vi "generate default line.vi"(8 "error in":errorcluster, 10 "last line":T1, 11 "operations table":T2) -> (0 "error out":errorcluster, 2 "line":T1)   [LabVIEW 2013, in "Modbus Slave editor node.lvclass"]
doc: "Platypus Framework 1.0.1.65\nNI Systems Engineering - National Instruments"
uses:
  Modbus Slave editor node.lvclass
  table line.ctl
  <vilib>/NI/Tag Bus/tag/tag descriptor.lvclass
  module/module channel/Modbus Module Channel.lvclass
  <vilib>/NI/Tag Bus/tag/Data Type.ctl
  module/module channel/data bank type.ctl
  table reference.ctl
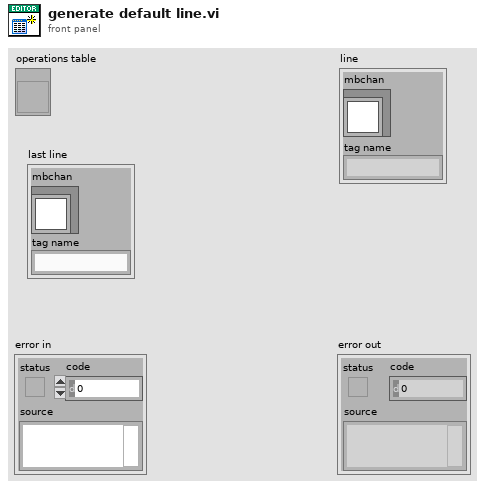
[diagram p1: front panel]
types:
  T1 = typedef "Modbus Slave editor node.lvclass/table line.ctl" = cluster{"mbchan":refnum<class "Modbus Module Channel.lvclass">, "tag name":string}
  T2 = typedef "Modbus Slave editor node.lvclass/table reference.ctl" = refnum<vi>
  T3 = typedef "tag bus.lvlib/tag descriptor.lvclass/Data Type.ctl" = enum16{"Double", "Single", "I64", "I32", "I16", "I8", "U64", "U32", "U16", "U8", "Boolean", "String", "Array of Double", "Array of Single", "Array of I64", "Array of I32", "Array of I16", "Array of I8", "Array of U64", "Array of U32", "Array of U16", "Array of U8", "Array of Boolean", "Array of String"}
  T4 = typedef "Modbus Module Channel.lvclass/data bank type.ctl" = enum16{"coils", "discrete inputs", "input registers", "holding registers"}
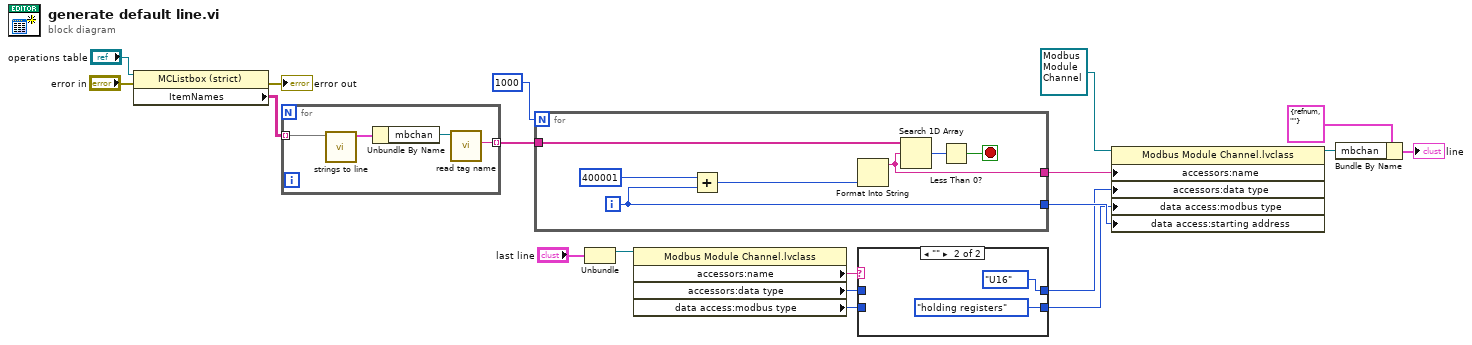
[diagram p0: block diagram]
diagram:
  n1 = property class="MCListbox (strict)"(reference="operations table", error in="error in") -> (error out=→"error out":errorcluster, "ItemNames"=w16:string[][])  [unwired: 1 out]
  n2 = for {
    tunnel: w16 -> [w23] mode=indexing
    tunnel: [w20] -> w14 mode=indexing
    n3 = call "strings to line.vi"("strings"=w23) -> ("line"=w22:T1)  [unwired: 10 in]
    n4 = Unbundle By Name(w22) -> ("mbchan"=w21:refnum<class "Modbus Module Channel.lvclass">)
    n5 = call <vilib>:"read tag name.vi"("system tag in"=w21) -> ("name"=w20:string)  [unwired: 8 in, 2 out]
  }
  n6 = for {
    N: 1000 -> [_]
    tunnel: w14 -> [w30]
    tunnel: [w27] -> w9
    tunnel: [w24] -> w8
    i -> [w24]
    stop <- w28 stop-if-true
    n7 = Add(x=400001, y=w24) -> (x+y=w26:i32)
    n8 = Format Into String(w26) -> (resulting string=w27:string)  [unwired: 3 in, 1 out]
    n9 = Search 1D Array(1D array=w30, element=w27) -> (index of element=w29:i32)  [unwired: 1 in]
    n10 = Less Than 0?(x=w29) -> (x < 0?=w28:bool)
  }
  n11 = Unbundle("last line") -> ("mbchan"=w6:refnum<class "Modbus Module Channel.lvclass">)  [unwired: 1 out]
  n12 = property class="Modbus Module Channel.lvclass"(reference=w6) -> ("accessors:name"=w5:string, "accessors:data type"=w2:T3, "data access:modbus type"=w1:T4)  [unwired: 1 in, 2 out]
  n13 = case shown="\"\"" w5 {
    tunnel: [w32 Data_Type."U16" ("data type")] -> w4
    tunnel: [w31 data_bank_type."holding registers" ("modbus type")] -> w3
    tunnel: w2 -> [w32 _]
    tunnel: w1 -> [w31 _]
    frame Default {
    }
    frame "" {
    }
  }
  n14 = property class="Modbus Module Channel.lvclass"(reference=refnum<class "Modbus Module Channel.lvclass"> refnum ("Modbus Module Channel"), "accessors:name"=w9, "accessors:data type"=w4, "data access:modbus type"=w3, "data access:starting address"=w8) -> (reference out=w10:refnum<class "Modbus Module Channel.lvclass">)  [unwired: 1 in, 1 out]
  n15 = Bundle By Name(cluster=T1 {"mbchan"=refnum, "tag name"=""} ("line"), "mbchan"=w10) -> (→"line":T1)
